vi "Basic Calculator.vi"() -> ()   [LabVIEW 2015]
panel:
  out "Answer":ext
  in  "Second":i32
  in  "First":i32
  in  "Operator":T1(ring)
  # ".."
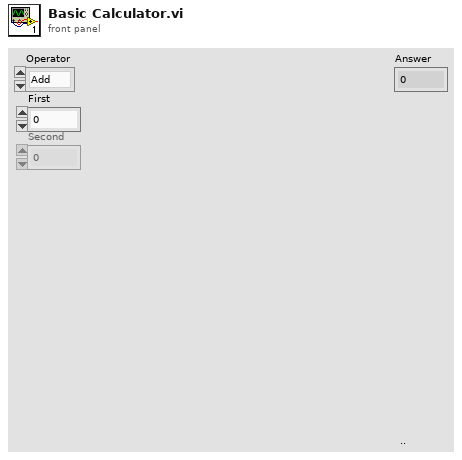
[diagram p1: front panel]
types:
  T1 = enum16{"Add", "Subtract", "Multiply", "Divide", "Square", "Root"}
  T2 = enum8{"Enabled", "Disabled", "Disabled and Grayed Out"}
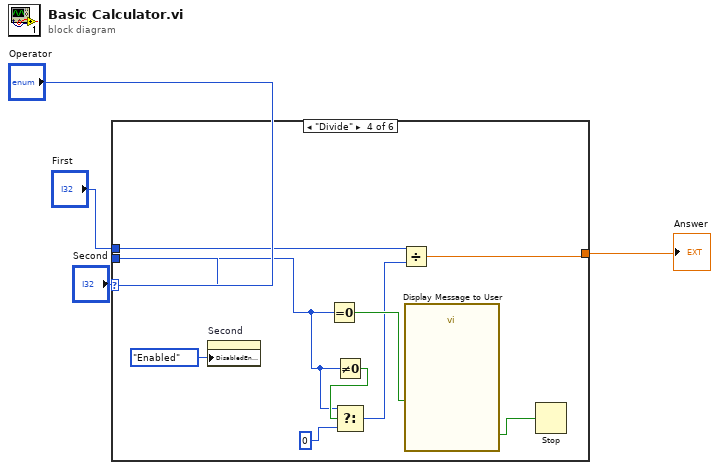
[diagram p0: block diagram]
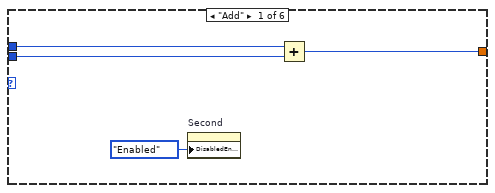
[diagram p2: hidden frame]
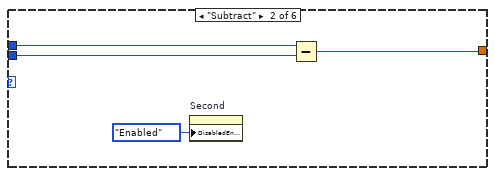
[diagram p3: hidden frame]
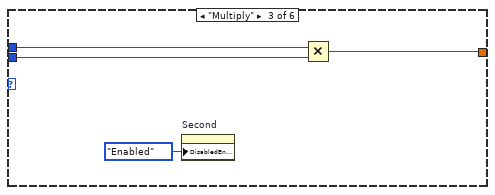
[diagram p4: hidden frame]
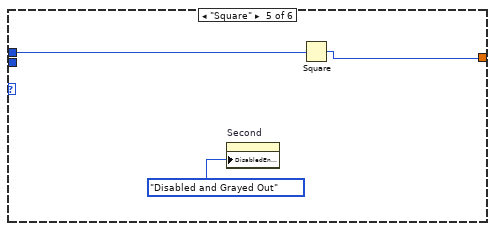
[diagram p5: hidden frame]
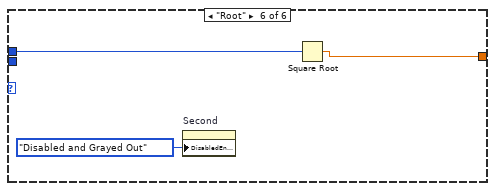
[diagram p6: hidden frame]
diagram:
  n1 = case shown="\"Divide\"" "Operator" {
    tunnel: "First" -> [w8 w12 w16 w25 w28 w31]
    tunnel: "Second" -> [w7 w11 w15 w21 _ _]
    tunnel: [w6 w10 w14 w24 w27 w30] -> w2
    frame "Add" {
      n2 = property on="Second" class="DigNum (strict)"("DisabledEnum"=T2."Enabled" ("Disabled")) -> ()  [unwired: 2 in, 2 out]
      n3 = Add(x=w8, y=w7) -> (x+y=w6:i32)
    }
    frame "Subtract" {
      n4 = property on="Second" class="DigNum (strict)"("DisabledEnum"=T2."Enabled" ("Disabled")) -> ()  [unwired: 2 in, 2 out]
      n5 = Subtract(x=w12, y=w11) -> (x-y=w10:i32)
    }
    frame "Multiply" {
      n6 = property on="Second" class="DigNum (strict)"("DisabledEnum"=T2."Enabled" ("Disabled")) -> ()  [unwired: 2 in, 2 out]
      n7 = Multiply(x=w16, y=w15) -> (x*y=w14:i32)
    }
    frame "Divide" {
      n8 = property on="Second" class="DigNum (strict)"("DisabledEnum"=T2."Enabled" ("Disabled")) -> ()  [unwired: 2 in, 2 out]
      n9 = Equal To 0?(x=w21) -> (x = 0?=w23:bool)
      n10 = Not Equal To 0?(x=w21) -> (x != 0?=w22:bool)
      n11 = Select(t=w21, s=w22, f=0) -> (s? t:f=w19:i32)
      n12 = Divide(x=w25, y=w19) -> (x/y=w24:dbl)
      n13 = call "Display Message to User"("Enable"=w23) -> ("OK"=w17:bool)  [unwired: 9 in, 1 out]
      n14 = Stop(stop? (T)=w17) -> ()
    }
    frame "Square" {
      n15 = property on="Second" class="DigNum (strict)"("DisabledEnum"=T2."Disabled and Grayed Out" ("Disabled")) -> ()  [unwired: 2 in, 2 out]
      n16 = Square(x=w28) -> (x^2=w27:i32)
    }
    frame "Root" {
      n17 = property on="Second" class="DigNum (strict)"("DisabledEnum"=T2."Disabled and Grayed Out" ("Disabled")) -> ()  [unwired: 2 in, 2 out]
      n18 = Square Root(x=w31) -> (sqrt(x)=w30:dbl)
    }
  }
  "Answer" <- w2
